vi "SMO Provider.vi"() -> (2 "Refs":refnum<vi>[](array[refnum]), 3 "SMOs":refnum<class "Test Helper 1.lvclass">[](array[class]))   [LabVIEW 2019]
uses:
  Helper/Test Helper 1/Test Helper 1.lvclass
  <vilib>/JKI/JKI SMO/SMO/SMO.lvclass
  Helper/Test Helper 2/Test Helper 2.lvclass
  Helper/Test Helper 3/Test Helper 3.lvclass
  C:/Program Files (x86)/National Instruments/LabVIEW 2020/vi.lib/JKI/JKI SMO/SMO/SMO.lvclass
  C:/Users/Patrick/Documents/GitHub/MAUI-Engine/lvsrc/Maui 2.0/Tests/Helper/Test Helper 1/Test Helper 1.lvclass
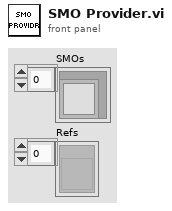
[diagram p1: front panel]
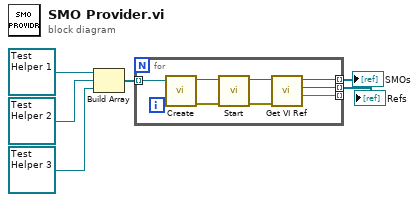
[diagram p0: block diagram]
diagram:
  n1 = Build Array(refnum<class "Test Helper 1.lvclass"> refnum ("Test Helper 1.lvclass"), refnum<class "Test Helper 2.lvclass"> refnum ("Test Helper 2.lvclass"), refnum<class "Test Helper 3.lvclass"> refnum ("Test Helper 3.lvclass")) -> (w3:refnum<class "Test Helper 1.lvclass">[])
  n2 = for {
    tunnel: w3 -> [w14] mode=indexing
    tunnel: [w10] -> w2 mode=indexing
    tunnel: [w9] -> w1 mode=indexing
    tunnel: [w8] -> _ mode=indexing
    n3 = call <vilib>:"Create.vi"("SMO"=w14) -> ("error out"=w12:errorcluster, "SMO out"=w13:refnum<class "Test Helper 1.lvclass">)  [unwired: 8 in, 1 out]
    n4 = call <vilib>:"Start.vi"("error in (no error)"=w12, "SMO"=w13) -> ("error out"=w7:errorcluster, "SMO out"=w11:refnum<class "Test Helper 1.lvclass">)  [unwired: 8 in]
    n5 = call-dynamic "Get VI Ref.vi"("error in (no error)"=w7, "Test Helper 1 in"=w11) -> ("VI Clone Name"=w8:string, "Static VI Ref"=w9:refnum<vi>, "Test Helper 1 out"=w10:refnum<class "Test Helper 1.lvclass">)  [unwired: 6 in, 1 out]
  }
  "SMOs" <- w2
  "Refs" <- w1
